vi "Cal BC (VIRef).vi"(8 "error in (no error)":errorcluster, 10 "BC in":variant, 11 "Domain_Evolut_2D_Rect in":refnum<class "NI_Domain_Evolut_2D_Rect.lvclass">) -> (0 "error out":errorcluster, 2 "BC out":variant, 3 "Domain_Evolut_2D_Rect out":refnum<class "NI_Domain_Evolut_2D_Rect.lvclass">)   [LabVIEW 2020, in "NI_PDE.lvlib" / "NI_Domain_Evolut_2D_Rect.lvclass"]
uses:
  <vilib>/gmath/pde.llb/DomainClass/Domain_Evolut_2D_Rect/NI_Domain_Evolut_2D_Rect.lvclass
  <vilib>/gmath/pde.llb/Common/PDE_BC Position 2D.ctl
  <vilib>/gmath/pde.llb/BCClass/BC_Evolut_2D_VIRef/BC Data.ctl
  <vilib>/gmath/pde.llb/Common/PDE_BC Type.ctl
  <vilib>/gmath/pde.llb/BCClass/BC_Evolut_2D_Numeric/BC Data.ctl
  <vilib>/gmath/pde.llb/DomainClass/Domain_Evolut_2D_Rect/NI_Domain_Evolut_2D_Rect.lvclass/NI_Domain_Evolut_2D_Rect.ctl
  <vilib>/Analysis/1siggen.llb/Ramp Pattern by Samples.vi
  <vilib>/gmath/NI_PDE.lvlib
  <vilib>/gmath/pde.llb/BCClass/BC_Evolut_2D_VIRef/NI_BC_Evolut_2D_VIRef.lvclass
  <vilib>/gmath/pde.llb/BCClass/BC_Evolut_2D_Numeric/NI_BC_Evolut_2D_Numeric.lvclass
  <vilib>/Analysis/NI_AALBase.lvlib
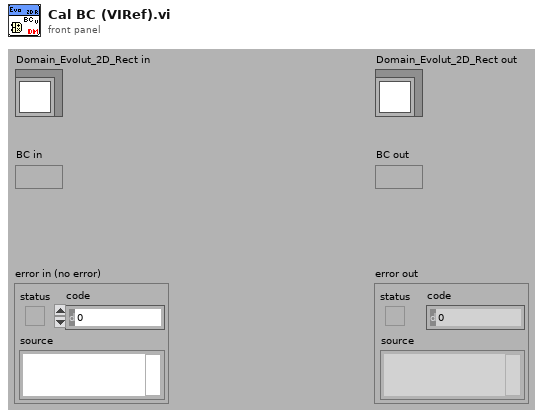
[diagram p1: front panel]
types:
  T1 = typedef "NI_PDE.lvlib/NI_BC_Evolut_2D_Numeric.lvclass/BC Data.ctl" = cluster{"type":T2, "position":T3, "G":dbl[][]}
  T2 = typedef "NI_PDE.lvlib/PDE_BC Type.ctl" = i32
  T3 = typedef "NI_PDE.lvlib/PDE_BC Position 2D.ctl" = i32
  T4 = typedef "NI_PDE.lvlib/NI_BC_Evolut_2D_VIRef.lvclass/BC Data.ctl" = cluster{"type":T2, "position":T3, "G":refnum<vi>, "data":variant}
  T5 = cluster{"initial t":dbl, "final t":dbl, "# of t-points":i32}
  T6 = cluster{"start x":dbl, "end x":dbl, "# of x-points":i32}
  T7 = cluster{"start y":dbl, "end y":dbl, "# of y-points":i32}
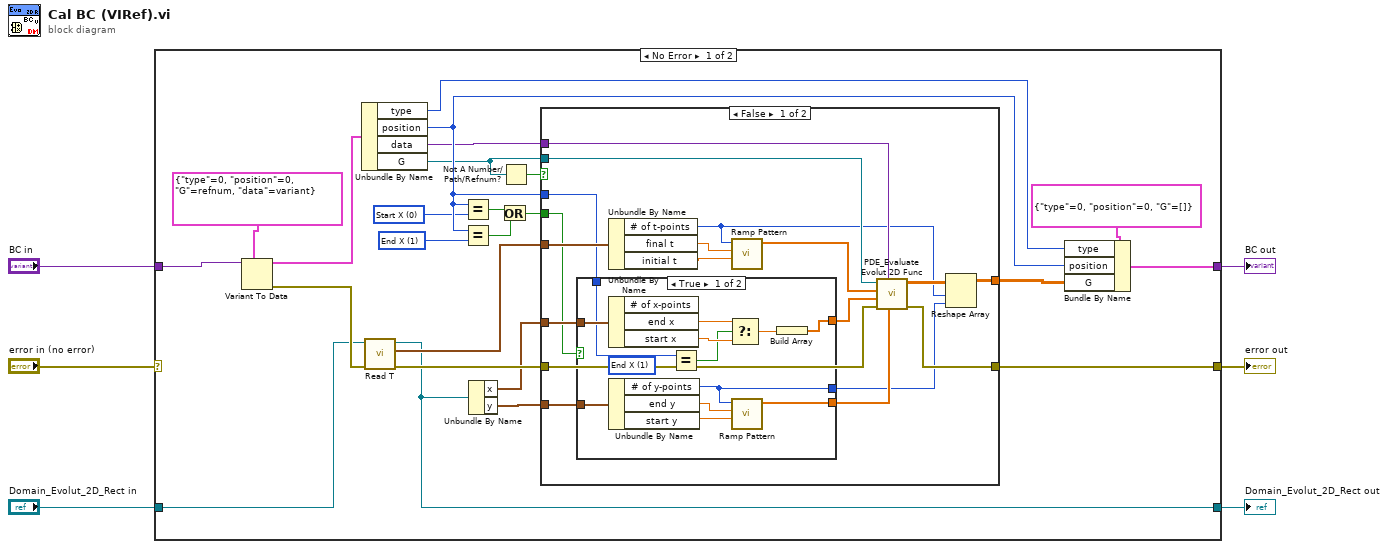
[diagram p0: block diagram]
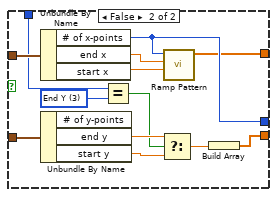
[diagram p2: hidden frame]
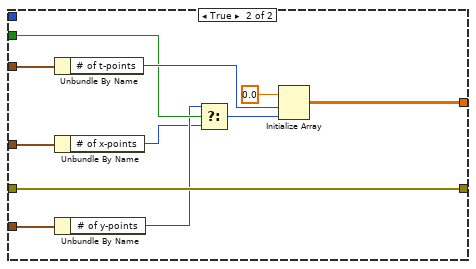
[diagram p3: hidden frame]
diagram:
  n1 = case shown="No Error" "error in (no error)" {
    selector: "error in (no error)" -> [_ w88]
    tunnel: "Domain_Evolut_2D_Rect in" -> [w10 w87]
    tunnel: [w7 w87] -> w6
    tunnel: [w11 w88] -> w5
    tunnel: [w14 w86] -> w2
    tunnel: "BC in" -> [w12 w86]
    frame No Error {
      w21 = T3 1 items=["Start X", "End X", "Start Y", "End Y"] ("y")
      w20 = T3 0 items=["Start X", "End X", "Start Y", "End Y"] ("y")
      n2 = Variant To Data(type=T4 {"type"=0, "position"=0, "G"=refnum, "data"=variant} ("BC data"), Variant=w12) -> (data=w27:T4, error out=w26:errorcluster)  [unwired: 1 in]
      n3 = Unbundle By Name(w27) -> ("type"=w29:T2, "position"=w30:T3, "data"=w19:variant, "G"=w18:refnum<vi>)
      n4 = call-dynamic "Read T.vi"("error in (no error)"=w26, "Domain_Evolut.lvclass in"=w10) -> ("error out"=w16:errorcluster, "t"=w15:T5, "Domain_Evolut.lvclass out"=w7:refnum<class "NI_Domain_Evolut_2D_Rect.lvclass">)  [unwired: 7 out]
      n5 = Equal?(x=w30, y=w20) -> (x = y?=w22:bool)
      n6 = Equal?(x=w30, y=w21) -> (x = y?=w23:bool)
      n7 = Unbundle By Name(w7) -> ("x"=w9:T6, "y"=w8:T7)
      n8 = Or(x=w22, y=w23) -> (x .or. y?=w24:bool)
      n9 = Not A Number/Path/Refnum?(number/path/refnum=w18) -> (NaN/Path/Refnum?=w17:bool)
      n10 = case shown="False" w17 {
        tunnel: [w31 w85] -> w13
        tunnel: w15 -> [w48 w84]
        tunnel: w16 -> [w39 w82]
        tunnel: [w47 w82] -> w11
        tunnel: w18 -> [w46 _]
        tunnel: w19 -> [w45 _]
        tunnel: w30 -> [w36 _]
        tunnel: w9 -> [w42 w79]
        tunnel: w8 -> [w34 w78]
        tunnel: w24 -> [w35 w80]
        frame False {
          n11 = case shown="True" w35 {
            tunnel: w42 -> [w61 w74]
            tunnel: [w60 w62] -> w40
            tunnel: w36 -> [w55 w72]
            tunnel: w34 -> [w54 w71]
            tunnel: [w50 w69] -> w33
            tunnel: [w49 w63] -> w32
            frame True {
              w56 = T3 1 items=["Start X", "End X", "Start Y", "End Y"] ("y")
              n12 = Unbundle By Name(w61) -> ("end x"=w59:dbl, "start x"=w58:dbl)  [unwired: 1 out]
              n13 = Unbundle By Name(w54) -> ("# of y-points"=w49:i32, "end y"=w52:dbl, "start y"=w51:dbl)
              n14 = Equal?(x=w55, y=w56) -> (x = y?=w53:bool)
              n15 = Select(t=w59, s=w53, f=w58) -> (s? t:f=w57:dbl)
              n16 = call-poly <vilib>:"Ramp Pattern.vi"("start"=w51, "end"=w52, "samples"=w49) -> ("Ramp Pattern"=w50:dbl[])  [unwired: 7 in, 1 out]
              n17 = Build Array(w57) -> (w60:dbl[])
            }
            frame False {
              w73 = T3 3 items=["Start X", "End X", "Start Y", "End Y"] ("y")
              n18 = Unbundle By Name(w74) -> ("# of x-points"=w63:i32, "end x"=w64:dbl, "start x"=w65:dbl)
              n19 = Unbundle By Name(w71) -> ("end y"=w68:dbl, "start y"=w67:dbl)  [unwired: 1 out]
              n20 = Equal?(x=w72, y=w73) -> (x = y?=w66:bool)
              n21 = Select(t=w68, s=w66, f=w67) -> (s? t:f=w70:dbl)
              n22 = call-poly <vilib>:"Ramp Pattern.vi"("start"=w65, "end"=w64, "samples"=w63) -> ("Ramp Pattern"=w62:dbl[])  [unwired: 7 in, 1 out]
              n23 = Build Array(w70) -> (w69:dbl[])
            }
          }
          n24 = Unbundle By Name(w48) -> ("# of t-points"=w43:i32, "final t"=w37:dbl, "initial t"=w38:dbl)
          n25 = call-poly <vilib>:"Ramp Pattern.vi"("start"=w38, "end"=w37, "samples"=w43) -> ("Ramp Pattern"=w41:dbl[])  [unwired: 7 in, 1 out]
          n26 = call <vilib>:"PDE_Evaluate Evolut 2D Func.vi"("Y"=w33, "data"=w45, "error in (no error)"=w39, "X"=w40, "T"=w41, "VIRef"=w46) -> ("error out"=w47:errorcluster, "F(t, x, y)"=w44:dbl[][][])  [unwired: 4 out]
          n27 = Reshape Array(w44, w43, w32) -> (w31:dbl[][])
        }
        frame True {
          n28 = Unbundle By Name(w84) -> ("# of t-points"=w81:i32)
          n29 = Unbundle By Name(w79) -> ("# of x-points"=w76:i32)
          n30 = Unbundle By Name(w78) -> ("# of y-points"=w77:i32)
          n31 = Select(t=w77, s=w80, f=w76) -> (s? t:f=w75:i32)
          n32 = Initialize Array(0.0 ("element"), w81, w75) -> (w85:dbl[][])
        }
      }
      n33 = Bundle By Name(cluster=T1 {"type"=0, "position"=0, "G"=[]} ("BC data"), "type"=w29, "position"=w30, "G"=w13) -> (w14:T1)
    }
    frame Error {
    }
  }
  "Domain_Evolut_2D_Rect out" <- w6
  "error out" <- w5
  "BC out" <- w2
